vi "Open Connection_Control 1.vi"(8 "error in (no error)":errorcluster, 9 "Cluster1":T1, 10 "topicName":string) -> (0 "error out":errorcluster, 3 "topicRef":cluster{"topicName":string, "type":refnum<vi>})   [LabVIEW 2012]
uses:
  SALTypedefs/Control 1.ctl
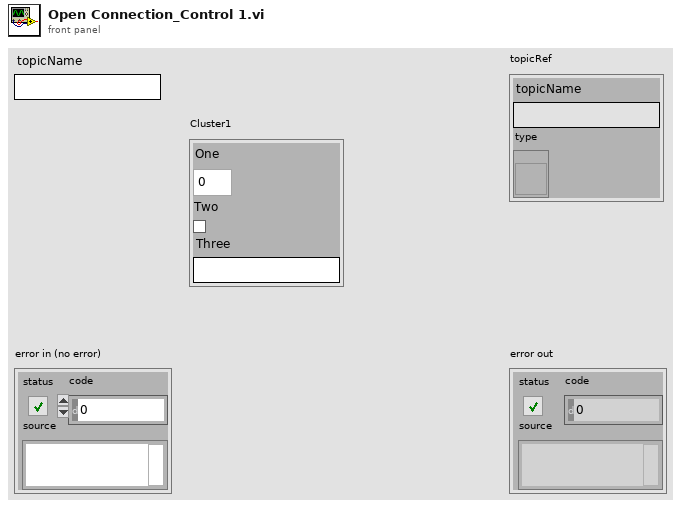
[diagram p1: front panel]
types:
  T1 = typedef "Control 1.ctl" = cluster{"One":dbl, "Two":bool, "Three":string}
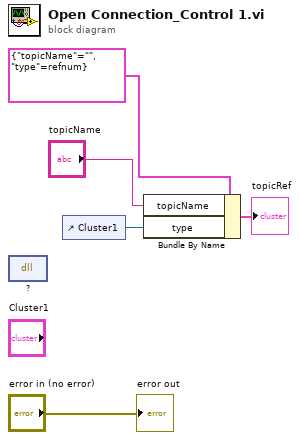
[diagram p0: block diagram]
diagram:
  n1 = dll-call lib="?" fn="?"() -> ()  [unwired: 4 in, 2 out]
  n2 = control-ref of="Cluster1"() -> (w2:refnum<vi>)
  n3 = Bundle By Name(cluster=cluster{"topicName":string, "type":refnum<vi>} {"topicName"="", "type"=refnum} ("topicRef"), "topicName"="topicName", "type"=w2) -> (→"topicRef":cluster{"topicName":string, "type":refnum<vi>})
  "error out" <- "error in (no error)"
